vi "Joystick interpolation.vi"() -> ()   [LabVIEW 2017]
uses:
  <vilib>/Analysis/1siggen.llb/Ramp Pattern by Delta.vi
  <vilib>/gmath/NI_Gmath.lvlib
  <vilib>/Analysis/NI_AALBase.lvlib
panel:
  in  "Numeric":dbl=1000.0 format="%#_13g"
  in  "method":i32(ring)=3 items=["nearest", "linear", "spline", "cubic Hermite", "Lagrange"]
  in  "Slide 5":dbl(slide) scale=0.0..1.0
  in  "Slide 6":dbl(slide) scale=0.0..1.0
  out "Power":dbl(slide) scale=-1.0..1.0
  in  "Joystick Sim":dbl(slide) scale=-1.0..1.0
  in  "Slide 4":dbl(slide) scale=0.0..1.0
  in  "Slide 3":dbl(slide) scale=0.0..1.0
  in  "Slide 2":dbl(slide) scale=0.0..1.0
  in  "Slide":dbl(slide) scale=0.0..1.0
  out "Interpolated Data":dbl[][](array[numeric])
  out "1D Interpolation Graph":cluster{"yi":dbl[], "ramp data":dbl[]}[](graph)
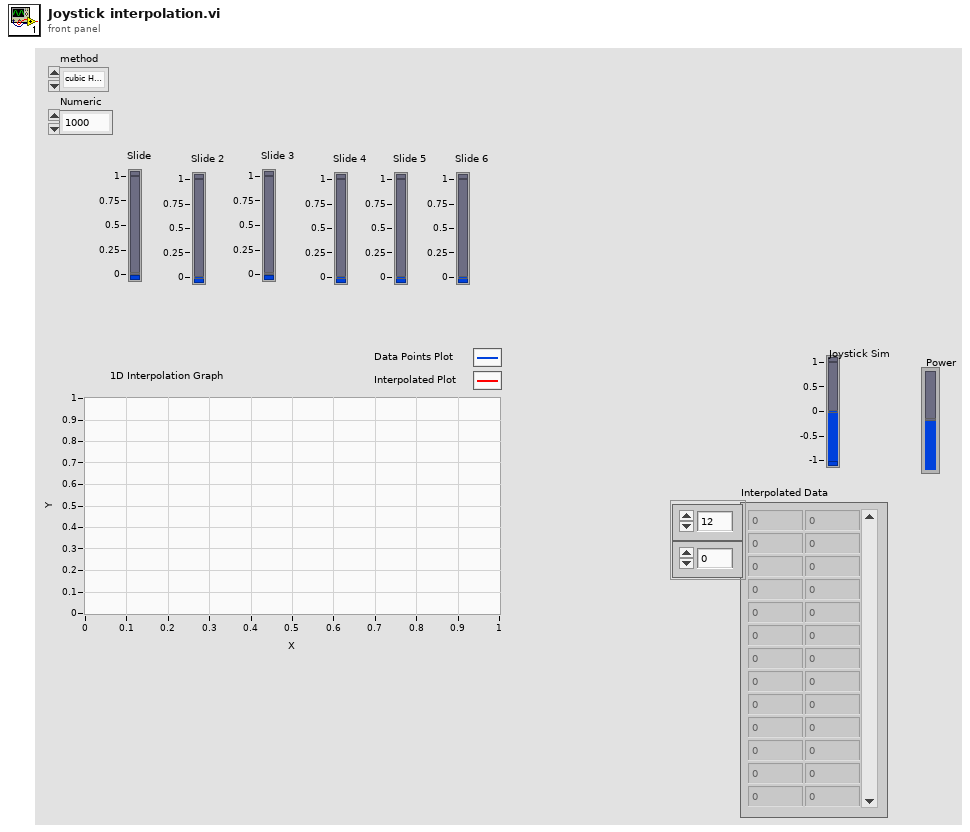
[diagram p1: front panel]
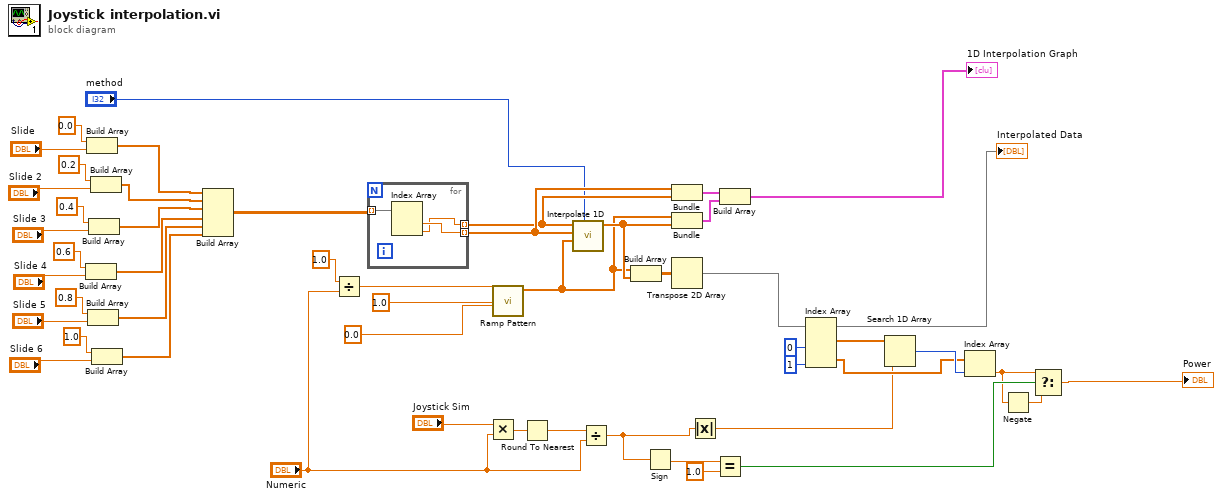
[diagram p0: block diagram]
diagram:
  n1 = Build Array(0.6 ("element"), "Slide 4") -> (w39:dbl[])
  n2 = Build Array(0.0 ("element"), "Slide") -> (w42:dbl[])
  n3 = Build Array(0.8 ("element"), "Slide 5") -> (w29:dbl[])
  n4 = Build Array(0.4 ("element"), "Slide 3") -> (w40:dbl[])
  n5 = Build Array(0.2 ("element"), "Slide 2") -> (w41:dbl[])
  n6 = Build Array(1.0 ("element"), "Slide 6") -> (w28:dbl[])
  n7 = Build Array(w42, w41, w40, w39, w29, w28) -> (w6:dbl[][])
  n8 = Divide(x=1.0 ("delta"), y="Numeric") -> (x/y=w1:dbl)
  n9 = for {
    tunnel: [w51] -> w13 mode=indexing
    tunnel: [w52] -> w14 mode=indexing
    tunnel: w6 -> [w53] mode=indexing
    n10 = Index Array(array=w53) -> (element #1=w52:dbl, element #2=w51:dbl)  [unwired: 2 in]
  }
  n11 = Multiply(x="Joystick Sim", y="Numeric") -> (x*y=w26:dbl)
  n12 = call-poly <vilib>:"Ramp Pattern.vi"("start"=0.0, "end"=1.0, "delta"=w1) -> ("Ramp Pattern"=w10:dbl[])  [unwired: 6 in, 2 out]
  n13 = Round To Nearest(number=w26) -> (nearest integer value=w25:dbl)
  n14 = call <vilib>:"Interpolate 1D.vi"("method"="method", "xi"=w10, "X"=w14, "Y"=w13) -> ("yi"=w11:dbl[])  [unwired: 5 in, 2 out]
  n15 = Divide(x=w25, y="Numeric") -> (x/y=w24:dbl)
  n16 = Build Array(w10, w11) -> (w12:dbl[][])
  n17 = Sign(1:w24) -> (0:w22:dbl)
  n18 = Bundle(w14, w13) -> (w15:cluster{dbl[], dbl[]})  [unwired: 1 in]
  n19 = Bundle("Ramp Pattern"=w10, "yi"=w11) -> (w16:cluster{"Ramp Pattern":dbl[], "yi":dbl[]})  [unwired: 1 in]
  n20 = Transpose 2D Array(2D array=w12) -> (transposed array=w4:dbl[][])
  "Interpolated Data" <- w4
  n21 = Absolute Value(x=w24) -> (abs(x)=w23:dbl)
  n22 = Equal?(x=w22, y=1.0) -> (x = y?=w20:bool)
  n23 = Build Array(w15, w16) -> (→"1D Interpolation Graph":cluster{"Ramp Pattern":dbl[], "yi":dbl[]}[])
  n24 = Index Array(array=w4, index (col) #1=0 ("disabled index (col)"), index (col) #2=1 ("index (col)")) -> (element #1=w34:dbl[], element #2=w35:dbl[])  [unwired: 2 in]
  n25 = Search 1D Array(1D array=w34, element=w23) -> (index of element=w38:i32)  [unwired: 1 in]
  n26 = Index Array(array=w35, index=w38) -> (element=w18:dbl)
  n27 = Negate(x=w18) -> (-x=w19:dbl)
  n28 = Select(t=w18, s=w20, f=w19) -> (s? t:f=→"Power":dbl)
